vi "generateBoards.vi"(10 "Array":i32[][][](array[numeric])) -> (2 "BingoBoards":refnum<class "BingoBoard.lvclass">[](array[class]))   [LabVIEW 2017, in "BingoBoard.lvclass"]
uses:
  BingoBoard.lvclass
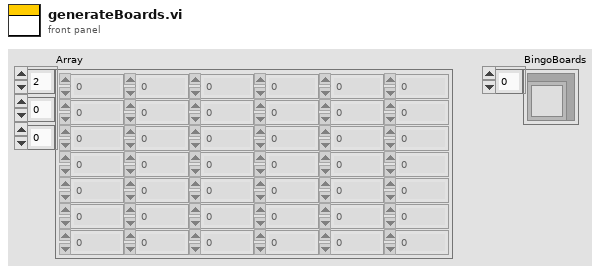
[diagram p1: front panel]
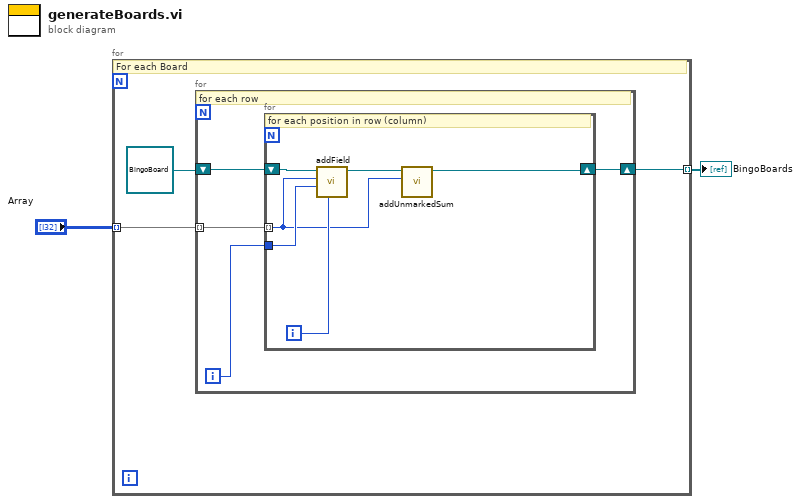
[diagram p0: block diagram]
diagram:
  n1 = for {
    tunnel: "Array" -> [w5] mode=indexing
    tunnel: [w3] -> w1 mode=indexing
    # "For each Board"
    n2 = for {
      tunnel: w5 -> [w9] mode=indexing
      shift-right: [w6] -> w3
      shift-left: refnum<class "BingoBoard.lvclass"> refnum ("BingoBoard.lvclass") -> [w7]
      i -> [w8]
      # "for each row"
      n3 = for {
        tunnel: w9 -> [w12] mode=indexing
        tunnel: w8 -> [w15]
        shift-right: [w10] -> w6
        shift-left: w7 -> [w13]
        i -> [w14]
        # "for each position in row (column)"
        n4 = call "addField.vi"("col"=w14, "row"=w15, "value"=w12, "BingoBoard in"=w13) -> ("BingoBoard out"=w11:refnum<class "BingoBoard.lvclass">)  [unwired: 7 in]
        n5 = call "addUnmarkedSum.vi"("Numeric"=w12, "BingoBoard in"=w11) -> ("output cluster"=w10:refnum<class "BingoBoard.lvclass">)  [unwired: 9 in]
      }
    }
  }
  "BingoBoards" <- w1
